vi "OpenIVIsampleswitch.vi"(0 "logical name (\"SampleSwitch\")":string="SampleSwitch") -> (1 "instrument handle":refnum<k15>, 2 "self test result":i16, 3 "self-test message":string, 4 "error in (no error)":errorcluster)   [LabVIEW 2010]
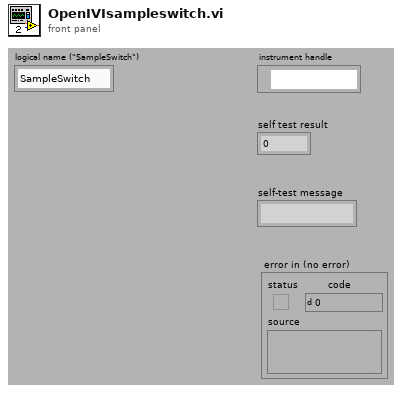
[diagram p1: front panel]
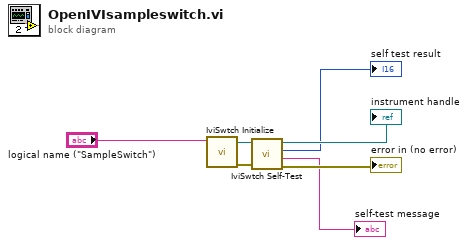
[diagram p0: block diagram]
diagram:
  n1 = call <vilib>:"IviSwtch Initialize.vi"("logical name (\"SampleSwitch\")"="logical name (\"SampleSwitch\")") -> ("error out"=w1:errorcluster, "instrument handle out"=w2:refnum<k15>)  [unwired: 3 in, 6 out]
  n2 = call <vilib>:"IviSwtch Self-Test.vi"("error in (no error)"=w1, "instrument handle"=w2) -> ("error out"=→"error in (no error)":errorcluster, "self-test message"=→"self-test message":string, "self test result"=→"self test result":i16, "instrument handle out"=→"instrument handle":refnum<k15>)  [unwired: 6 out]
